vi "RUSHShoot.vi"(1 "In Cluster":T2) -> (0 "Out Cluster":T1)   [LabVIEW 2012]
panel:
  out "ShootOutIndexer":dbl
  out "ShootOutElev":dbl
  out "ShootOutCase":dbl
  out "ShootOutWheelF":dbl
  out "ShootOutWheelB":dbl
  in  "ShootPOTToPowConst":dbl=0.2
  in  "Shooter WheelB Spd Const":dbl=0.7
  in  "Shooter WheelF Spd Const":dbl=0.7
  in  "Indexer Spd Const":dbl=0.5
  in  "Vision Speed Const":dbl=0.75
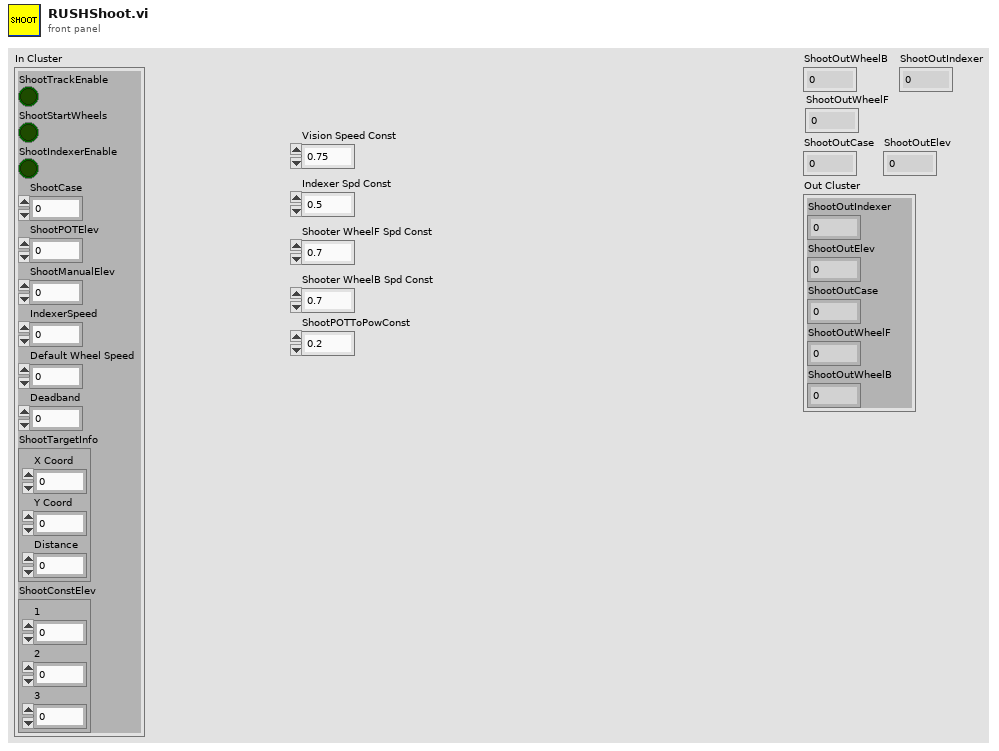
[diagram p1: front panel]
types:
  T1 = cluster{"ShootOutIndexer":dbl, "ShootOutElev":dbl, "ShootOutCase":dbl, "ShootOutWheelF":dbl, "ShootOutWheelB":dbl}
  T2 = cluster{"ShootTrackEnable":bool, "ShootStartWheels":bool, "ShootIndexerEnable":bool, "ShootCase":dbl, "ShootPOTElev":dbl, "ShootManualElev":dbl, "IndexerSpeed":dbl, "Default Wheel Speed":dbl, "Deadband":dbl, "ShootTargetInfo":cluster{"X Coord":dbl, "Y Coord":dbl, "Distance":dbl}, "ShootConstElev":cluster{"1":dbl, "2":dbl, "3":dbl}}
  T3 = cluster{"X Coord":dbl, "Y Coord":dbl, "Distance":dbl}
  T4 = cluster{"f":dbl, "upper limit":dbl, "upper limit":dbl, "f":dbl, "f":dbl}
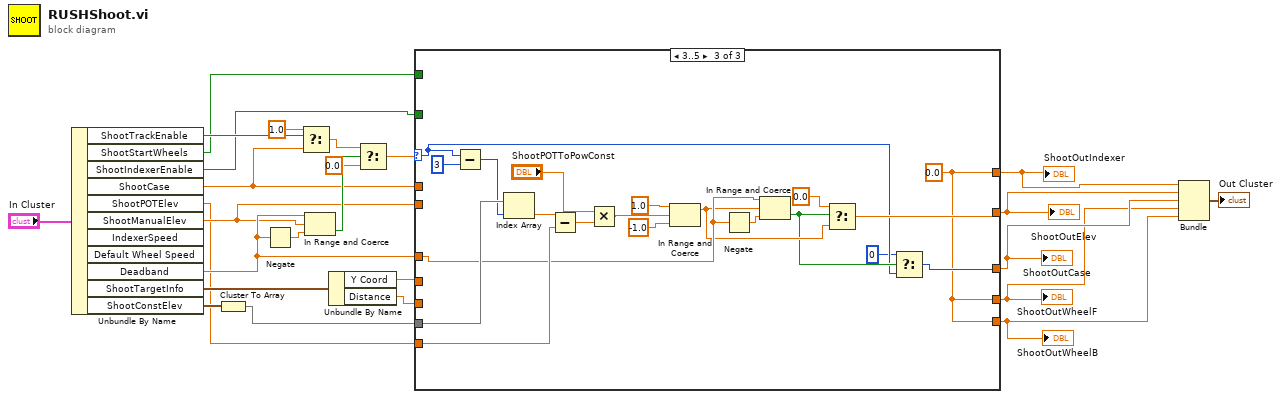
[diagram p0: block diagram]
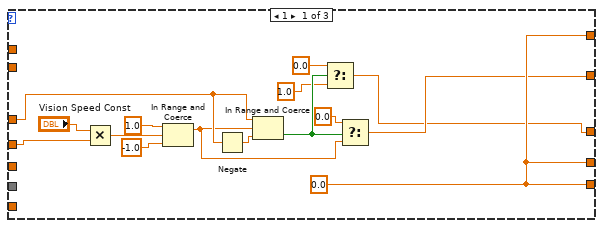
[diagram p2: hidden frame]
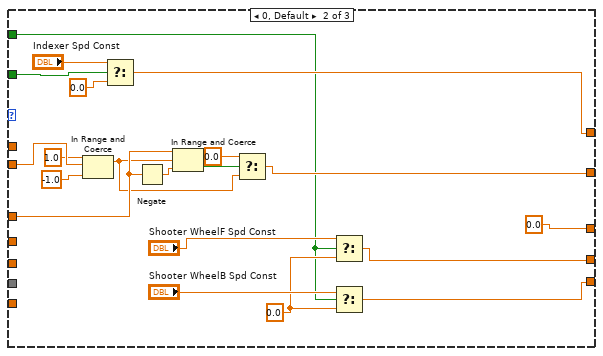
[diagram p3: hidden frame]
diagram:
  n1 = Unbundle By Name("In Cluster") -> ("ShootTrackEnable"=w24:bool, "ShootStartWheels"=w12:bool, "ShootIndexerEnable"=w11:bool, "ShootCase"=w13:dbl, "ShootPOTElev"=w7:dbl, "ShootManualElev"=w10:dbl, "Deadband"=w14:dbl, "ShootTargetInfo"=w17:T3, "ShootConstElev"=w9:cluster{"1":dbl, "2":dbl, "3":dbl})  [unwired: 2 out]
  n2 = Cluster To Array(cluster=w9) -> (array=w8:dbl[])
  n3 = Negate(x=w14) -> (-x=w21:dbl)
  n4 = Select(t=1.0, s=w24, f=w13) -> (s? t:f=w22:dbl)
  n5 = In Range and Coerce(upper limit=w14, x=w10, lower limit=w21) -> (In Range?=w20:bool)  [unwired: 1 out]
  n6 = Unbundle By Name(w17) -> ("Y Coord"=w16:dbl, "Distance"=w15:dbl)
  n7 = Select(t=w22, s=w20, f=0.0) -> (s? t:f=w18:dbl)
  n8 = case shown="3..5" w18 {
    selector: w18 -> [_ _ w64]
    tunnel: w16 -> [w39 _ _]
    tunnel: w15 -> [_ _ _]
    tunnel: w14 -> [w34 w53 w69]
    tunnel: [w27 0.0 ("upper limit") w62] -> w4
    tunnel: w13 -> [_ _ _]
    tunnel: [w28 w49 w66] -> w5
    tunnel: [w29 w43 w61] -> w2
    tunnel: [w29 w44 w61] -> w3
    tunnel: [w29 w57 w61] -> w6
    tunnel: w12 -> [_ w45 _]
    tunnel: w11 -> [_ w59 _]
    tunnel: w10 -> [_ w54 _]
    tunnel: w8 -> [_ _ w79]
    tunnel: w7 -> [_ _ w76]
    frame 1 {
      w29 = 0.0
      n9 = Multiply(x="Vision Speed Const", y=w39) -> (x*y=w38:dbl)
      n10 = In Range and Coerce(upper limit=1.0, x=w38, lower limit=-1.0 ("upper limit")) -> (coerced(x)=w32:dbl)  [unwired: 1 out]
      n11 = Negate(x=w34) -> (-x=w35:dbl)
      n12 = In Range and Coerce(upper limit=w34, x=w32, lower limit=w35) -> (In Range?=w31:bool)  [unwired: 1 out]
      n13 = Select(t=0.0, s=w31, f=1.0) -> (s? t:f=w27:dbl)
      n14 = Select(t=0.0, s=w31, f=w32) -> (s? t:f=w28:dbl)
    }
    frame 0, Default {
      w46 = 0.0 ("t")
      n15 = In Range and Coerce(upper limit=1.0, x=w54, lower limit=-1.0 ("upper limit")) -> (coerced(x)=w50:dbl)  [unwired: 1 out]
      n16 = Select(t="Indexer Spd Const", s=w59, f=0.0) -> (s? t:f=w57:dbl)
      n17 = Negate(x=w53) -> (-x=w55:dbl)
      n18 = In Range and Coerce(upper limit=w53, x=w50, lower limit=w55) -> (In Range?=w52:bool)  [unwired: 1 out]
      n19 = Select(t=0.0, s=w52, f=w50) -> (s? t:f=w49:dbl)
      n20 = Select(t="Shooter WheelF Spd Const", s=w45, f=w46) -> (s? t:f=w44:dbl)
      n21 = Select(t="Shooter WheelB Spd Const", s=w45, f=w46) -> (s? t:f=w43:dbl)
    }
    frame 3..5 {
      w61 = 0.0 ("f")
      n22 = Subtract(x=w64, y=3) -> (x-y=w78:i32)
      n23 = Index Array(array=w79, index=w78) -> (element=w77:dbl)
      n24 = Subtract(x=w77, y=w76) -> (x-y=w75:dbl)
      n25 = Multiply(x="ShootPOTToPowConst", y=w75) -> (x*y=w70:dbl)
      n26 = In Range and Coerce(upper limit=1.0, x=w70, lower limit=-1.0 ("upper limit")) -> (coerced(x)=w67:dbl)  [unwired: 1 out]
      n27 = Negate(x=w69) -> (-x=w71:dbl)
      n28 = In Range and Coerce(upper limit=w69, x=w67, lower limit=w71) -> (In Range?=w65:bool)  [unwired: 1 out]
      n29 = Select(t=0.0, s=w65, f=w67) -> (s? t:f=w66:dbl)
      n30 = Select(t=0, s=w65, f=w64) -> (s? t:f=w62:i32)
    }
  }
  "ShootOutWheelB" <- w2
  "ShootOutWheelF" <- w3
  "ShootOutCase" <- w4
  "ShootOutElev" <- w5
  "ShootOutIndexer" <- w6
  n31 = Bundle("f"=w6, "upper limit"=w5, "upper limit"=w4, "f"=w3, "f"=w2) -> (→"Out Cluster":T4)  [unwired: 1 in]
